vi "Render Variable.vi"(8 "Error In":errorcluster, 10 "Tag":refnum<class "Variable.lvclass">, 11 "Context In":refnum<class "Context.lvclass">) -> (0 "Error Out":errorcluster, 2 "Output":string, 3 "Context Out":refnum<class "Context.lvclass">)   [LabVIEW 2018, in "Toolkit.lvlib"]
uses:
  Toolkit.lvlib
  Nodes/Variable/Variable.lvclass
  Context/Context.lvclass
  Nodes/Variable/Variable.lvclass/Variable.ctl
  Data/String/String.lvclass
  Data/String/String.lvclass/String.ctl
  Data/Datum/Datum.lvclass
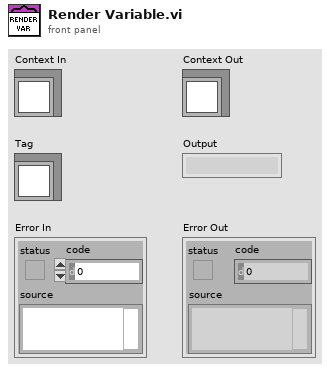
[diagram p1: front panel]
types:
  T1 = typedef "Toolkit.lvlib/Data.lvlib/Types.ctl" = enum16{"Array", "Boolean", "Function", "Map", "Null", "Path", "String", "Unknown"}
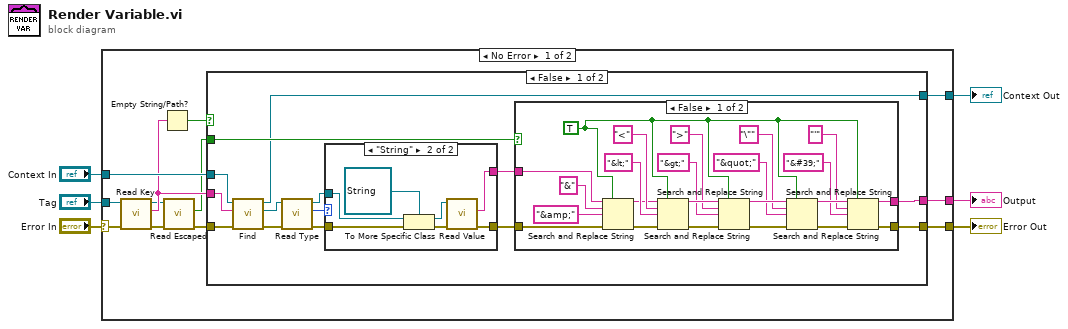
[diagram p0: block diagram]
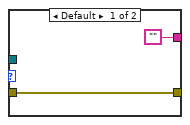
[diagram p2: hidden frame]
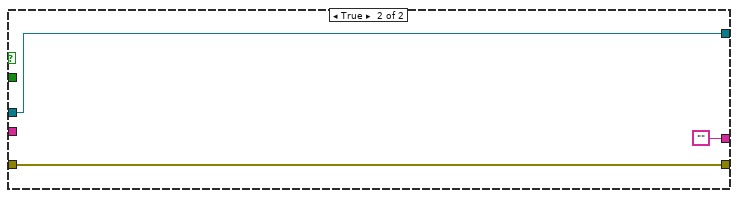
[diagram p4: hidden frame]
diagram:
  n1 = case shown="No Error" "Error In" {
    selector: "Error In" -> [w13 w71]
    tunnel: "Tag" -> [w12 _]
    tunnel: [w18 w71] -> w4
    tunnel: [w17 _] -> w3
    tunnel: "Context In" -> [w16 w70]
    tunnel: [w14 w70] -> w1
    frame No Error {
      n2 = call "Read Key.vi"("Error In"=w13, "Variable In"=w12) -> ("Error Out"=w9:errorcluster, "Key"=w11:string, "Variable Out"=w10:refnum<class "Variable.lvclass">)  [unwired: 7 in]
      n3 = Empty String/Path?(string/path=w11) -> (empty?=w15:bool)
      n4 = call "Read Escaped.vi"("Error In"=w9, "Variable In"=w10) -> ("Error Out"=w7:errorcluster, "Escaped"=w8:bool)  [unwired: 7 in, 1 out]
      n5 = case shown="False" w15 {
        tunnel: [w32 w69] -> w18
        tunnel: [w31 ""] -> w17
        tunnel: w8 -> [w30 _]
        tunnel: w16 -> [w27 w67]
        tunnel: w11 -> [w26 _]
        tunnel: w7 -> [w25 w69]
        tunnel: [w23 w67] -> w14
        frame False {
          n6 = call "Find.vi"("Error In"=w25, "Key"=w26, "Context In"=w27) -> ("Error Out"=w21:errorcluster, "Datum"=w24:refnum<class "Datum.lvclass">, "Context Out"=w23:refnum<class "Context.lvclass">)  [unwired: 5 in, 1 out]
          n7 = call-dynamic "Read Type.vi"("Error In"=w21, "Datum In"=w24) -> ("Error Out"=w19:errorcluster, "Type"=w20:T1, "Datum Out"=w22:refnum<class "Datum.lvclass">)  [unwired: 7 in]
          n8 = case shown="\"String\"" w20 {
            tunnel: w19 -> [w34 w41]
            tunnel: w22 -> [_ w39]
            tunnel: [w34 w36] -> w29
            tunnel: ["" w35] -> w28
            frame Default {
            }
            frame "String" {
              n9 = To More Specific Class(target class=refnum<class "String.lvclass"> refnum ("Toolkit.lvlib:Data.lvlib:String.lvclass"), reference=w39, error in=w41) -> (specific class reference=w37:refnum<class "String.lvclass">, error out=w38:errorcluster)
              n10 = call "Read Value.vi"("Error In"=w38, "String In"=w37) -> ("Error Out"=w36:errorcluster, "Value"=w35:string)  [unwired: 7 in, 1 out]
            }
          }
          n11 = case shown="False" w30 {
            tunnel: [w45 w65] -> w32
            tunnel: [w44 w66] -> w31
            tunnel: w29 -> [w43 w65]
            tunnel: w28 -> [w42 w66]
            frame False {
              w48 = TRUE ("replace all? (F)")
              n12 = Search and Replace String(replace all?=w48, input string=w42, search string="&", replace string="&amp;" ("replace string (\"\")"), error in=w43) -> (result string=w60:string, error out=w59:errorcluster)  [unwired: 3 in, 2 out]
              n13 = Search and Replace String(replace all?=w48, input string=w60, search string="<", replace string="&lt;" ("replace string (\"\")"), error in=w59) -> (result string=w57:string, error out=w58:errorcluster)  [unwired: 3 in, 2 out]
              n14 = Search and Replace String(replace all?=w48, input string=w57, search string=">", replace string="&gt;" ("replace string (\"\")"), error in=w58) -> (result string=w53:string, error out=w54:errorcluster)  [unwired: 3 in, 2 out]
              n15 = Search and Replace String(replace all?=w48, input string=w53, search string="\"" ("replace string (\"\")"), replace string="&quot;" ("replace string (\"\")"), error in=w54) -> (result string=w50:string, error out=w49:errorcluster)  [unwired: 3 in, 2 out]
              n16 = Search and Replace String(replace all?=w48, input string=w50, search string="'", replace string="&#39;" ("replace string (\"\")"), error in=w49) -> (result string=w44:string, error out=w45:errorcluster)  [unwired: 3 in, 2 out]
            }
            frame True {
            }
          }
        }
        frame True {
        }
      }
    }
    frame Error {
    }
  }
  "Error Out" <- w4
  "Output" <- w3
  "Context Out" <- w1
